vi "write_params.vi"(8 "error in (no error)":errorcluster, 10 "params":T1={"C"=1.0, "fit_intercept"=TRUE, "max_iter"=1000.0, "tol"={"tol_type"="", "tol_float"=0.001}, "early_stopping"=FALSE, "validation_fraction"=0.1, "n_iter_no_change"=5.0, "shuffle"=TRUE, "verbose"=0.0, "loss"="epsilon_insensitive", "epsilon"=0.1, "random_state"=0.0, "warm_start"=FALSE, "average"=FALSE}, 11 "PassiveAggressiveRegressor in":refnum<class "PassiveAggressiveRegressor.lvclass">) -> (0 "error out":errorcluster, 3 "PassiveAggressiveRegressor out":refnum<class "PassiveAggressiveRegressor.lvclass">)   [LabVIEW 2020, in "PassiveAggressiveRegressor.lvclass"]
uses:
  PassiveAggressiveRegressor.lvclass
  Controls/passive_agressive_regressor_params.ctl
  PassiveAggressiveRegressor.lvclass/PassiveAggressiveRegressor.ctl
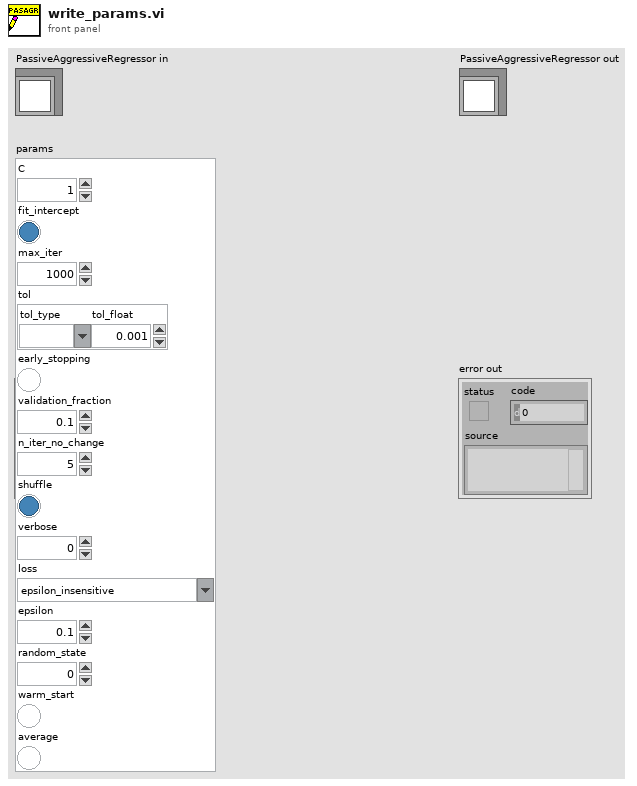
[diagram p1: front panel]
types:
  T1 = typedef "passive_agressive_regressor_params.ctl" = cluster{"C":dbl, "fit_intercept":bool, "max_iter":dbl, "tol":cluster{"tol_type":string, "tol_float":dbl}, "early_stopping":bool, "validation_fraction":dbl, "n_iter_no_change":dbl, "shuffle":bool, "verbose":dbl, "loss":string, "epsilon":dbl, "random_state":dbl, "warm_start":bool, "average":bool}
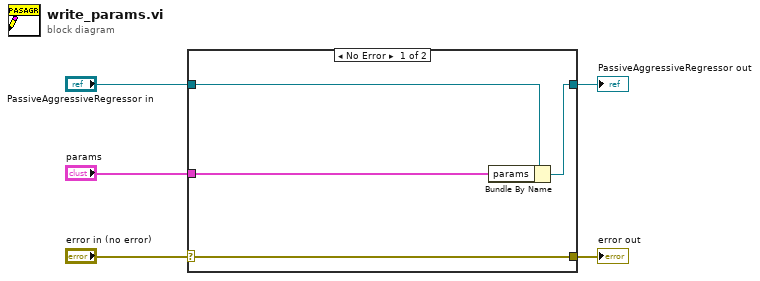
[diagram p0: block diagram]
diagram:
  n1 = case shown="No Error" "error in (no error)" {
    selector: "error in (no error)" -> [w9 w10]
    tunnel: [w9 w10] -> w4
    tunnel: [w7 w11] -> w2
    tunnel: "PassiveAggressiveRegressor in" -> [w8 w11]
    tunnel: "params" -> [w6 _]
    frame No Error {
      n2 = Bundle By Name(cluster=w8, "params"=w6) -> (w7:refnum<class "PassiveAggressiveRegressor.lvclass">)
    }
    frame Error {
    }
  }
  "error out" <- w4
  "PassiveAggressiveRegressor out" <- w2
